vi "Tegam4040 -- Get DLL Path.vi"(2 "DLL Path (system32)":enum16{"system32", "Debug", "Release", "Close"}(ring)) -> (7 "DLL Path":path)   [LabVIEW 2010]
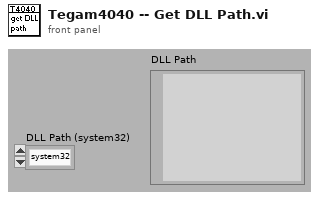
[diagram p1: front panel]
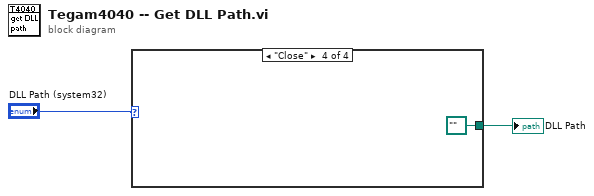
[diagram p0: block diagram]
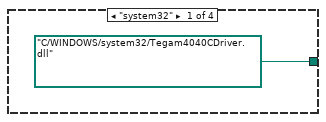
[diagram p2: hidden frame]
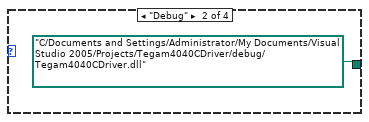
[diagram p3: hidden frame]
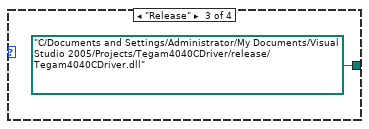
[diagram p4: hidden frame]
diagram:
  n1 = case shown="\"Close\"" "DLL Path (system32)" {
    tunnel: [path "C:/WINDOWS/system32/Tegam4040CDriver.dll" ("DLL Path") path "C:/Documents and Settings/Administrator/My Documents/Visual Studio 2005/Projects/Tegam4040CDriver/debug/Tegam4040CDriver.dll" ("DLL Path") path "C:/Documents and Settings/Administrator/My Documents/Visual Studio 2005/Projects/Tegam4040CDriver/release/Tegam4040CDriver.dll" ("DLL Path") path "" ("DLL Path")] -> w1
    frame "system32" {
    }
    frame "Debug" {
    }
    frame "Release" {
    }
    frame "Close" {
    }
  }
  "DLL Path" <- w1
